vi "Test Reference Harmonic.vi"(8 "error in (no error)":errorcluster, 11 "VISA resource name":refnum<visa-resource-name>) -> (0 "error out":errorcluster, 3 "VISA resource name":refnum<visa-resource-name>)   [LabVIEW 2019, in "SR7270 Drivers.lvlib"]
uses:
  SR7270 Drivers.lvlib
  Typedefs/REFMODE--enum.ctl
  Typedefs/VRLOCK--enum.ctl
  <userlib>/_OpenG.lib/numeric/numeric.llb/Random Number Within Range - DBL__ogtk.vi
  <vilib>/addons/_JKI Toolkits/Caraya/classes/Assert/Assert.lvclass
  <vilib>/addons/_JKI Toolkits/Caraya/classes/Test/Test.lvclass
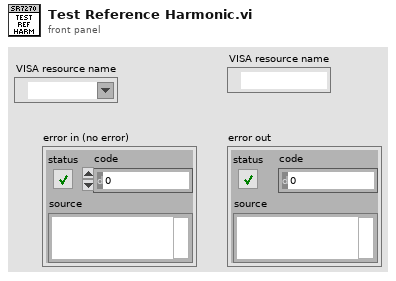
[diagram p1: front panel]
types:
  T1 = typedef "SR7270 Drivers.lvlib/VRLOCK--enum.ctl" = enum16{"Disabled", "Enabled"}
  T2 = typedef "SR7270 Drivers.lvlib/REFMODE--enum.ctl" = enum16{"Single Reference/Virtual Reference", "Dual Harmonic", "Dual Reference"}
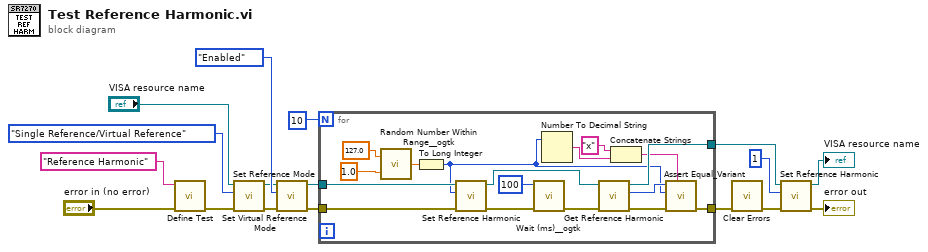
[diagram p0: block diagram]
diagram:
  n1 = call <vilib>:"Define Test.vi"("error in (no error)"="error in (no error)", "Label (VI Title)"="Reference Harmonic") -> ("error out"=w6:errorcluster)  [unwired: 9 in]
  n2 = call "Set Reference Mode.vi"("error in (no error)"=w6, "Reference Mode"=REFMODE--enum."Single Reference/Virtual Reference", "VISA resource name"="VISA resource name") -> ("error out"=w8:errorcluster, "VISA resource name out"=w5:refnum<visa-resource-name>)  [unwired: 7 in]
  n3 = call "Set Virtual Reference Mode.vi"("error in (no error)"=w8, "Virtual Reference Lock"=VRLOCK--enum."Enabled", "VISA resource name"=w5) -> ("error out"=w3:errorcluster, "VISA resource name out"=w4:refnum<visa-resource-name>)  [unwired: 7 in]
  n4 = for {
    N: 10 -> [_]
    tunnel: w4 -> [w33]
    tunnel: w3 -> [w26]
    tunnel: [w31] -> w17
    tunnel: [w30] -> w11
    n5 = call-poly <userlib>:"Random Number Within Range__ogtk.vi"("High"=127.0, "Low"=1.0) -> ("Random Number"=w22:dbl)  [unwired: 3 in]
    n6 = To Long Integer(number=w22) -> (32bit integer=w21:i32)
    n7 = call "Set Reference Harmonic.vi"("error in (no error)"=w26, "Harmonic"=w21, "VISA resource name"=w33) -> ("error out"=w27:errorcluster, "VISA resource name out"=w34:refnum<visa-resource-name>)  [unwired: 7 in]
    n8 = call <userlib>:"Wait (ms)__ogtk.vi"("error in (no error)"=w27, "milliseconds to wait"=u32 100) -> ("error out"=w29:errorcluster)  [unwired: 8 in, 1 out]
    n9 = Number To Decimal String(number=w21) -> (decimal integer string=w20:string)  [unwired: 1 in]
    n10 = call "Get Reference Harmonic.vi"("error in (no error)"=w29, "VISA resource name"=w34) -> ("error out"=w32:errorcluster, "Harmonic"=w25:i32, "VISA resource name out"=w30:refnum<visa-resource-name>)  [unwired: 7 in]
    n11 = Concatenate Strings("x" ("string"), w20) -> (w19:string)
    n12 = call <vilib>:"Assert Equal_Variant.vi"("Label"=w19, "error in (no error)"=w32, "Y"=w21, "X"=w25) -> ("error out"=w31:errorcluster)  [unwired: 7 in]
  }
  n13 = call <vilib>:"Clear Errors.vi"("error in (no error)"=w17) -> ("error out"=w13:errorcluster)  [unwired: 5 in, 1 out]
  n14 = call "Set Reference Harmonic.vi"("error in (no error)"=w13, "Harmonic"=1, "VISA resource name"=w11) -> ("error out"=→"error out":errorcluster, "VISA resource name out"=→"VISA resource name":refnum<visa-resource-name>)  [unwired: 7 in]
